vi "Pack Winbounds.vi"(3 "Front Panel.WinBounds":T1) -> (1 "value":string)   [LabVIEW 2015, in "User Interface.lvlib"]
uses:
  User Interface.lvlib
  <vilib>/Utility/miscctls.llb/LVRectTypeDef.ctl
  Error Correction/Error Correction.lvlib
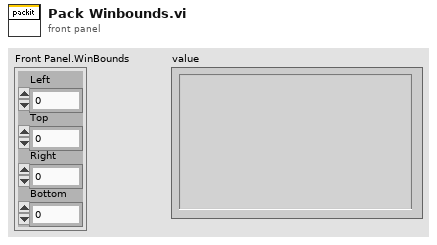
[diagram p1: front panel]
types:
  T1 = typedef "LVRectTypeDef.ctl" = cluster{"Left":i16, "Top":i16, "Right":i16, "Bottom":i16}
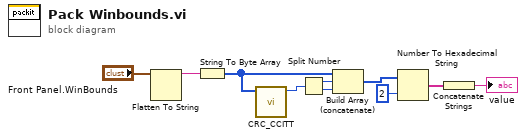
[diagram p0: block diagram]
diagram:
  n1 = Flatten To String(anything="Front Panel.WinBounds") -> (data string=w9:string)  [unwired: 3 in, 2 out]
  n2 = String To Byte Array(string=w9) -> (unsigned byte array=w5:u8[])
  n3 = call "CRC_CCITT.vi"("unsigned byte array"=w5) -> ("CRC-CCITT"=w3:u16)  [unwired: 5 in, 1 out]
  n4 = Split Number(x=w3) -> (hi(x)=w2:u8, lo(x)=w1:u8)
  n5 = Build Array (concatenate)(w5, w2, w1) -> (w4:u8[])
  n6 = Number To Hexadecimal String(1:i16 2 ("width (-)"), 2:w4) -> (0:w7:string[])
  n7 = Concatenate Strings(w7) -> (→"value":string)
